vi "VeriStand DSF.Transfer Group.Configuration.Create.vi"(8 "error in (no error)":errorcluster, 11 "Section Ref":T1=18446744073709551615 format="%.0x") -> (0 "error out":errorcluster, 3 "Transfer Group Configuration":refnum<class "VeriStand DSF.Transfer Group.Configuration.lvclass">)   [LabVIEW 2017, in "Data Sharing Framework Engine.lvlib" / "VeriStand DSF.Transfer Group.Configuration.lvclass"]
uses:
  VeriStand DSF.Transfer Group.Configuration.lvclass
  DSF Core/Built/Windows/Engine/DSF.Engine.lvlibp/Shared/Classes/Transfer Group/DSF.Shared.Configuration.Transfer Group.lvclass
  <vilib>/NI Veristand/Custom Device API/Custom Device API.lvlib
  VeriStand DSF.Transfer.Configuration.lvclass
  C:/Git/DSF/DSF Core/Built/Windows/Engine/DSF.Engine.lvlibp/Shared/Classes/Transfer/DSF.Shared.Configuration.Transfer.lvclass
  C:/Git/DSF/DSF Core/Built/Windows/Engine/DSF.Engine.lvlibp/Shared/Classes/Configuration/DSF.Shared.Configuration.lvclass
  C:/Git/DSF/DSF Core/Built/Windows/Engine/DSF.Engine.lvlibp/Shared/Classes/Transfer Group/DSF.Shared.Configuration.Transfer Group.lvclass
  <vilib>/NI Veristand/Custom Device API/Custom Device Item Ref.ctl
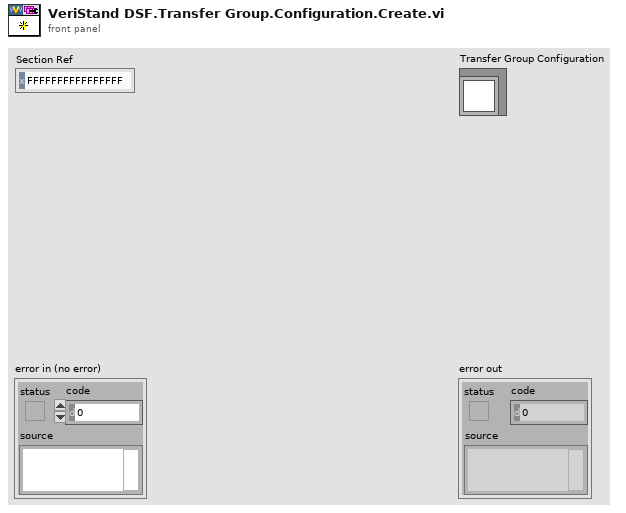
[diagram p1: front panel]
types:
  T1 = typedef "Custom Device API.lvlib/Custom Device Item Ref.ctl" = u64
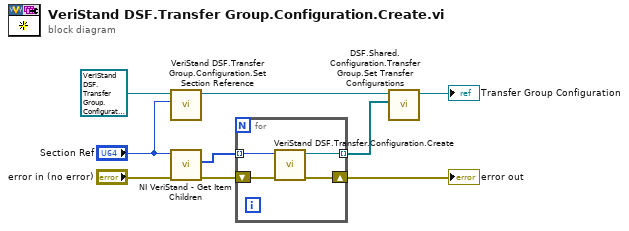
[diagram p0: block diagram]
diagram:
  n1 = call "VeriStand DSF.Transfer Group.Configuration.Set Section Reference.vi"("Section Ref"="Section Ref", "VeriStand DSF.Transfer Group.Configuration in"=refnum<class "VeriStand DSF.Transfer Group.Configuration.lvclass"> refnum ("VeriStand DSF.Plugin.Configuration in")) -> ("VeriStand DSF.Transfer Group.Configuration out"=w4:refnum<class "VeriStand DSF.Transfer Group.Configuration.lvclass">)  [unwired: 9 in]
  n2 = call <vilib>:"NI VeriStand - Get Item Children.vi"("error in (no error)"="error in (no error)", "Item Ref in"="Section Ref") -> ("error out"=w6:errorcluster, "Child Refs"=w5:T1[])  [unwired: 6 in, 2 out]
  n3 = for {
    tunnel: w5 -> [w12] mode=indexing
    tunnel: [w11] -> w3 mode=indexing
    shift-right: [w10] -> w1
    shift-left: w6 -> [w13]
    n4 = call "VeriStand DSF.Transfer.Configuration.Create.vi"("error in (no error)"=w13, "Section Ref"=w12) -> ("error out"=w10:errorcluster, "Transfer Configuration"=w11:refnum<class "VeriStand DSF.Transfer.Configuration.lvclass">)  [unwired: 8 in]
  }
  "error out" <- w1
  n5 = call "DSF.Shared.Configuration.Transfer Group.Set Transfer Configurations.vi"("Transfer Configurations"=w3, "Transfer Group Configuration in"=w4) -> ("Transfer Group Configuration out"=→"Transfer Group Configuration":refnum<class "VeriStand DSF.Transfer Group.Configuration.lvclass">)  [unwired: 9 in]
